vi "CU_trainCommittee.vi"(6 "DataTypes":T1, 8 "error in (no error)":errorcluster, 9 "Indices":i8[](array[numeric]), 11 "ClassifierClass in":refnum<class "ClassifierClass.lvclass">) -> (0 "error out":errorcluster, 1 "Classification Distribution":i32[][][](array[numeric]), 2 "Classifier Refs out":T2[](array[typedef]), 3 "ClassifierClass out":refnum<class "ClassifierClass.lvclass">)   [LabVIEW 2016, in "Classifier.lvlib" / "ClassifierClass.lvclass"]
uses:
  ClassifierClass.lvclass
  <vilib>/vision/Classification.llb/IMAQ Classifier Session.ctl
  CU_DataTypes.ctl
  ClassifierClass.lvclass/ClassifierClass.ctl
  <vilib>/vision/NI_Vision_Development_Module.lvlib
  Classifier.lvlib
panel:
  # "This VI is a part of BCI Design library, http://www.ru-bci.org \nCopyright © 2020, Sotnikov Peter, All rights reserved. License: GNU GPLv3"
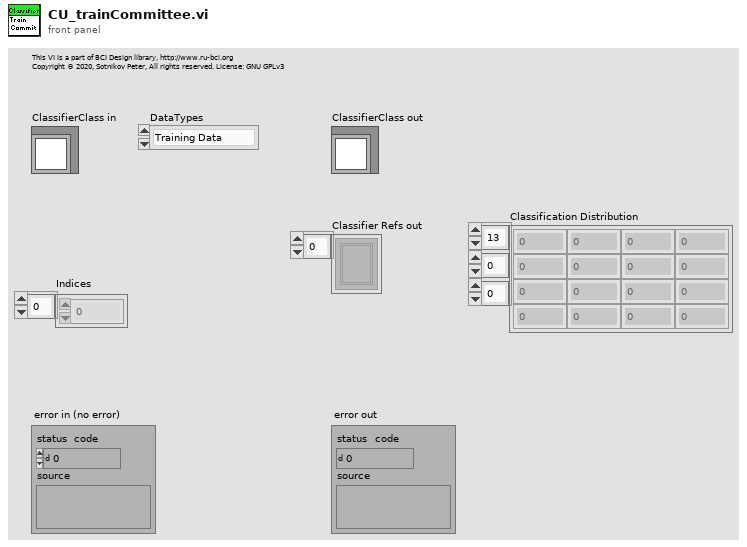
[diagram p1: front panel]
types:
  T1 = typedef "Classifier.lvlib/CU_DataTypes.ctl" = enum16{"Training Data", "Test Data", "Training Data (cross-check)", "Test Data (cross-check)"}
  T2 = typedef "IMAQ Classifier Session.ctl" = refnum<k1>
  T3 = typedef "XML_EEG_Features.lvlib/XML_FF_Trial.ctl" = cluster{"ClassLabel":string, "FeatureVector":dbl[]}
  T4 = typedef "IMAQ SVM Kernel Options.ctl" = cluster{"Kernel":enum32{"Linear", "Polynomial", "Gaussian", "RBF"}, "Degree":i32, "Gamma":dbl, "Coefficient":dbl, "Sigma":dbl, "Cache(MB)":dbl}
  T5 = typedef "IMAQ SVM Model Options.ctl" = cluster{"SVM Model":enum32{"C-SVC", "nu-SVC", "One Class"}, "Tolerance":dbl, "Max. Iteration":i32, "Nu":dbl, "Shrinking":bool, "Cost":dbl, "Weighted Cost":cluster{"Label":string, "Weight":dbl}[]}
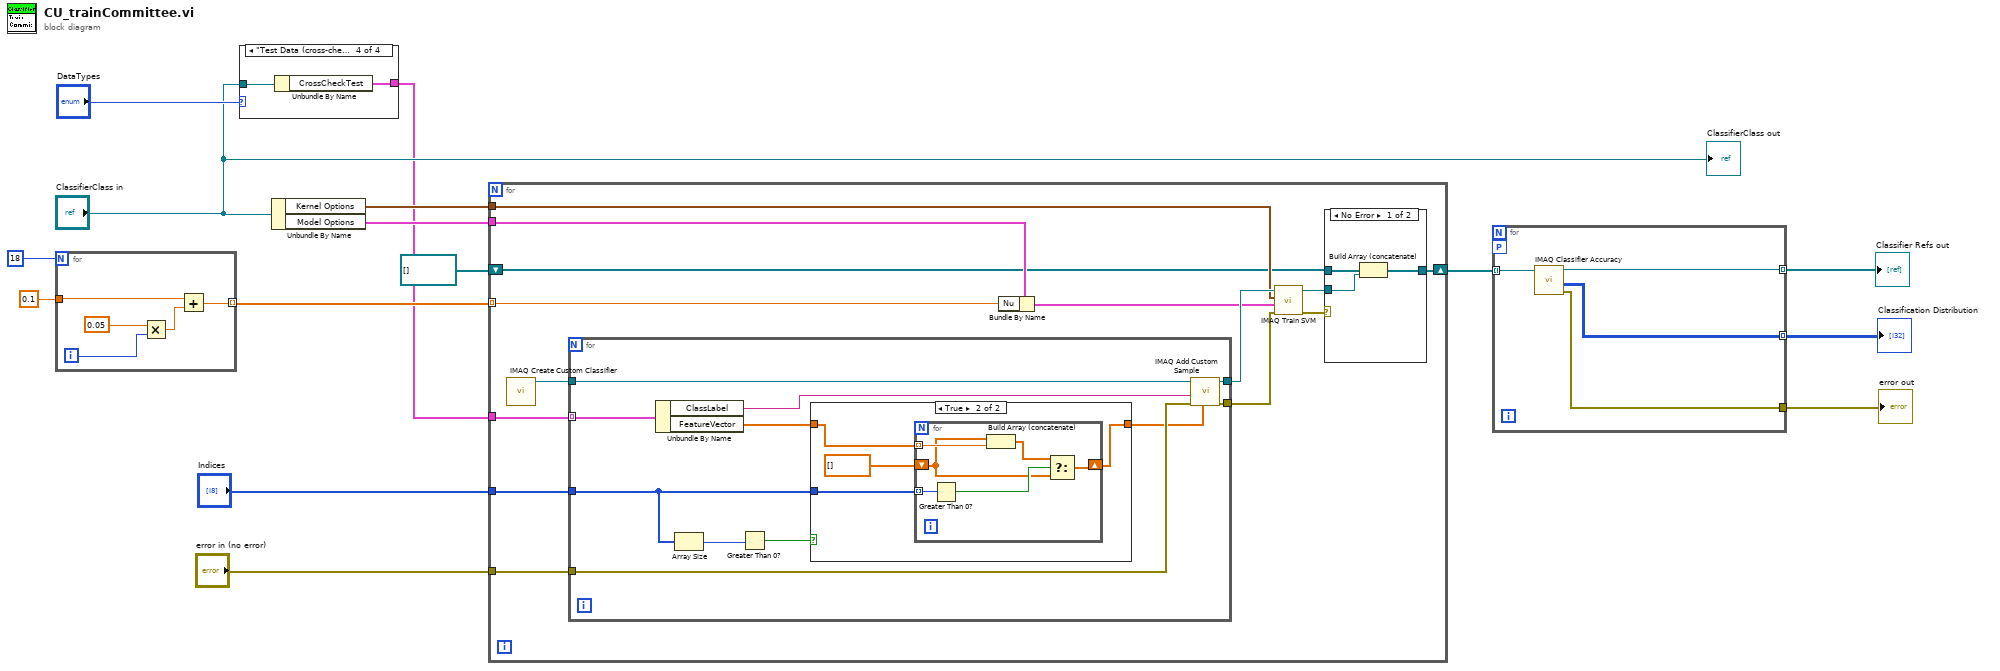
[diagram p0: block diagram]
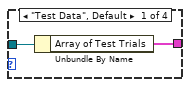
[diagram p2: hidden frame]
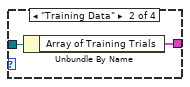
[diagram p3: hidden frame]
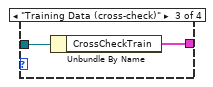
[diagram p4: hidden frame]
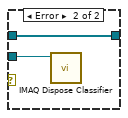
[diagram p5: hidden frame]
diagram:
  n1 = for {
    N: 18 -> [_]
    tunnel: 0.1 -> [w18]
    tunnel: [w16] -> w8 mode=indexing
    i -> [w17]
    n2 = Multiply(x=0.05, y=w17) -> (x*y=w19:dbl)
    n3 = Add(x=w18, y=w19) -> (x+y=w16:dbl)
  }
  n4 = case shown="\"Test Data (cross-check)\"" "DataTypes" {
    tunnel: "ClassifierClass in" -> [w22 w24 w26 w28]
    tunnel: [w21 w23 w25 w27] -> w1
    frame "Test Data", Default {
      n5 = Unbundle By Name(w22) -> ("Array of Test Trials"=w21:T3[])
    }
    frame "Training Data" {
      n6 = Unbundle By Name(w24) -> ("Array of Training Trials"=w23:T3[])
    }
    frame "Training Data (cross-check)" {
      n7 = Unbundle By Name(w26) -> ("CrossCheckTrain"=w25:T3[])
    }
    frame "Test Data (cross-check)" {
      n8 = Unbundle By Name(w28) -> ("CrossCheckTest"=w27:T3[])
    }
  }
  n9 = Unbundle By Name("ClassifierClass in") -> ("Kernel Options"=w13:T4, "Model Options"=w12:T5)
  n10 = for {
    tunnel: w1 -> [w42]
    tunnel: "error in (no error)" -> [w41]
    tunnel: "Indices" -> [w40]
    tunnel: w13 -> [w36]
    tunnel: w12 -> [w35]
    shift-right: [w32] -> w7
    shift-left: T2[] [] ("Classifier Refs out") -> [w31]
    tunnel: w8 -> [w30] mode=indexing
    n11 = call "IMAQ Create Custom Classifier"() -> ("Classifier Session"=w37:T2)  [unwired: 10 in, 1 out]
    n12 = for {
      tunnel: w42 -> [w58] mode=indexing
      tunnel: w37 -> [w57]
      tunnel: w41 -> [w55]
      tunnel: w40 -> [w50]
      tunnel: [w49] -> w39
      tunnel: [w48] -> w38
      n13 = Unbundle By Name(w58) -> ("ClassLabel"=w56:string, "FeatureVector"=w52:dbl[])
      n14 = Array Size(array=w50) -> (size(s)=w54:i32)
      n15 = Greater Than 0?(x=w54) -> (x > 0?=w53:bool)
      n16 = case shown="True" w53 {
        tunnel: w52 -> [w59 w63]
        tunnel: [w59 w60] -> w51
        tunnel: w50 -> [_ w62]
        frame False {
        }
        frame True {
          n17 = for {
            tunnel: w63 -> [w66] mode=indexing
            tunnel: w62 -> [w69] mode=indexing
            shift-right: [w68] -> w60
            shift-left: dbl[] [] -> [w64]
            n18 = Greater Than 0?(x=w69) -> (x > 0?=w67:bool)
            n19 = Build Array (concatenate)(w64, w66) -> (w65:dbl[])
            n20 = Select(t=w65, s=w67, f=w64) -> (s? t:f=w68:dbl[])
          }
        }
      }
      n21 = call "IMAQ Add Custom Sample"("Feature Vector"=w51, "error in (no error)"=w55, "Class"=w56, "Classifier Session"=w57) -> ("error out"=w49:errorcluster, "Classifier Session (dup)"=w48:T2)  [unwired: 6 in]
    }
    n22 = Bundle By Name(cluster=w35, "Nu"=w30) -> (w34:T5)
    n23 = call "IMAQ Train SVM"("error in (no error)"=w39, "Model Options"=w34, "Kernel Options"=w36, "Classifier Session"=w38) -> ("error out"=w33:errorcluster, "Classifier Session (dup)"=w29:T2)  [unwired: 4 in, 2 out]
    n24 = case shown="No Error" w33 {
      tunnel: [w43 w46] -> w32
      tunnel: w31 -> [w45 w46]
      tunnel: w29 -> [w44 w47]
      frame No Error {
        n25 = Build Array (concatenate)(w45, w44) -> (w43:T2[])
      }
      frame Error {
        n26 = call "IMAQ Dispose Classifier"("Classifier Session"=w47) -> ()  [unwired: 10 in, 1 out]
      }
    }
  }
  n27 = for {
    tunnel: w7 -> [w73] mode=indexing
    tunnel: [w70] -> w4 mode=indexing
    tunnel: [w72] -> w6 mode=indexing
    tunnel: [w71] -> w5
    workers-P: _ -> [_]
    n28 = call "IMAQ Classifier Accuracy"("Classifier Session"=w73) -> ("error out"=w71:errorcluster, "Classification Distribution"=w70:i32[][], "Classifier Session (dup)"=w72:T2)  [unwired: 4 in, 4 out]
  }
  "error out" <- w5
  "Classifier Refs out" <- w6
  "Classification Distribution" <- w4
  "ClassifierClass out" <- "ClassifierClass in"
